vi "Set CAN Publishing.vi"(5 "Box ID":u8=1, 7 "DIO":bool, 8 "error in (no error)":errorcluster, 9 "AI":bool, 10 "AO":bool, 11 "CAN in":refnum<class "XNET_BS120x.lvclass">) -> (0 "error out":errorcluster, 3 "CAN out":refnum<class "XNET_BS120x.lvclass">)   [LabVIEW 2021, in "BS120x Driver.lvlib" / "XNET_BS120x.lvclass"]
doc: "Configures which auxiliary I/O the Battery Simulator 1200 should publish. Used to reduce latency on CAN bus.\n(c) 2019 Bloomy Controls, Inc. All rights reserved."
uses:
  XNET_BS120x.lvclass
  BS120x.lvclass
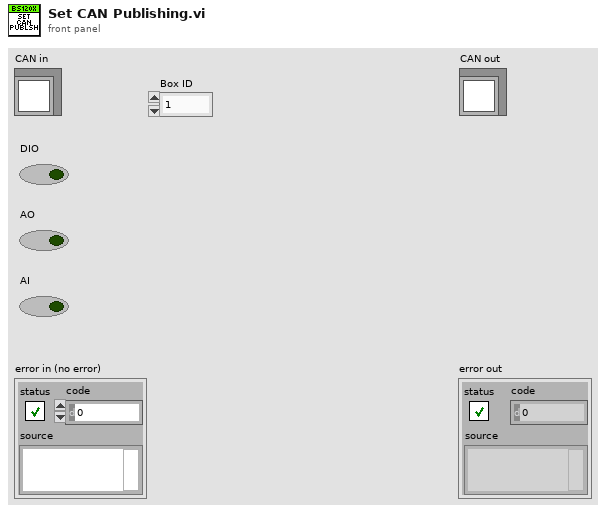
[diagram p1: front panel]
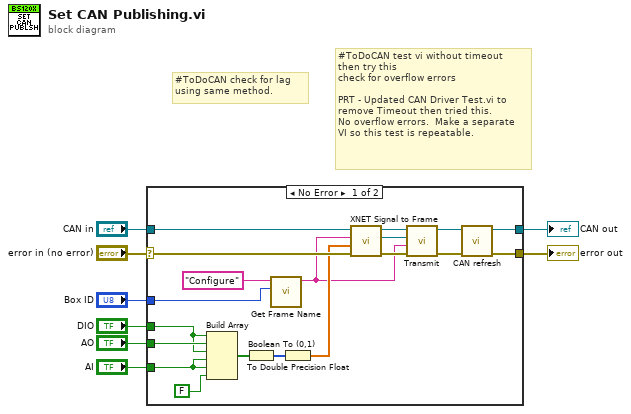
[diagram p0: block diagram]
diagram:
  # "#ToDoCAN check for lag\nusing same method."
  # "#ToDoCAN test vi without timeout\nthen try this\ncheck for overflow errors\n\nPRT - Updated CAN Driver Test.vi to\nremove Timeout then tried this.\nNo overflow errors.  Make a separate\nVI so this test is repeatable."
  n1 = case shown="No Error" "error in (no error)" {
    selector: "error in (no error)" -> [w26 w29]
    tunnel: [w20 w29] -> w7
    tunnel: [w18 w28] -> w5
    tunnel: "CAN in" -> [w25 w28]
    tunnel: "AI" -> [w13 _]
    tunnel: "AO" -> [w12 _]
    tunnel: "DIO" -> [w11 _]
    tunnel: "Box ID" -> [w16 _]
    frame No Error {
      n2 = Build Array(w11, w12, w11, w13, w13, FALSE ("element")) -> (w15:bool[])
      n3 = Boolean To (0,1)(Boolean=w15) -> (0, 1=w27:i16[])
      n4 = call "Get Frame Name.vi"("Box ID"=w16, "Frame Name"="Configure" ("name")) -> ("Frame Name out"=w9:string)  [unwired: 9 in]
      n5 = To Double Precision Float(number=w27) -> (double precision float=w14:dbl[])
      n6 = call "XNET Signal to Frame.vi"("error in (no error)"=w26, "Data Array"=w14, "Frame"=w9, "CAN in"=w25) -> ("error out"=w24:errorcluster, "Data"=w23:refnum<class "XNET Data.lvclass">, "CAN out"=w22:refnum<class "XNET_BS120x.lvclass">)  [unwired: 5 in]
      n7 = call "Transmit.vi"("error in (no error)"=w24, "Frame"=w9, "Data in"=w23, "CAN in"=w22) -> ("error out"=w21:errorcluster, "CAN out"=w19:refnum<class "XNET_BS120x.lvclass">)  [unwired: 6 in]
      n8 = call "CAN refresh.vi"("error in (no error)"=w21, "CAN in"=w19) -> ("error out"=w20:errorcluster, "CAN out"=w18:refnum<class "XNET_BS120x.lvclass">)  [unwired: 8 in]
    }
    frame Error {
    }
  }
  "error out" <- w7
  "CAN out" <- w5
